vi "Get State.vi"(8 "error in (no error)":errorcluster, 11 "Dual Relay Bricklet in":refnum<class "Dual Relay Bricklet.lvclass">) -> (0 "error out":errorcluster, 1 "relay 2":bool, 2 "relay 1":bool, 3 "Dual Relay Bricklet out":refnum<class "Dual Relay Bricklet.lvclass">)   [LabVIEW 2011, in "Tinkerforge.lvlib" / "Dual Relay Bricklet.lvclass"]
doc: "This VI returns the state of both relays."
uses:
  Dual Relay Bricklet.lvclass
  Type Definitions/Relay States.ctl
  Device/Device.lvclass
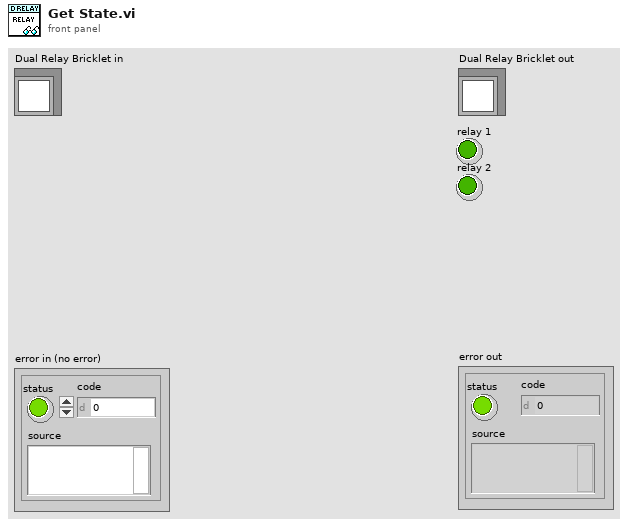
[diagram p1: front panel]
types:
  T1 = typedef "Tinkerforge.lvlib/Dual Relay Bricklet.lvclass/Relay States.ctl" = cluster{"relay 1":bool, "relay 2":bool}
  T2 = typedef "Tinkerforge.lvlib/IP Connection.lvclass/Answer.ctl" = cluster{"Request GUID":string, "Request Type":T3, "Sucessful":bool, "Data":variant, "Error":errorcluster}
  T3 = typedef "Tinkerforge.lvlib/IP Connection.lvclass/Request Type.ctl" = enum8{"Invalid", "Write"}
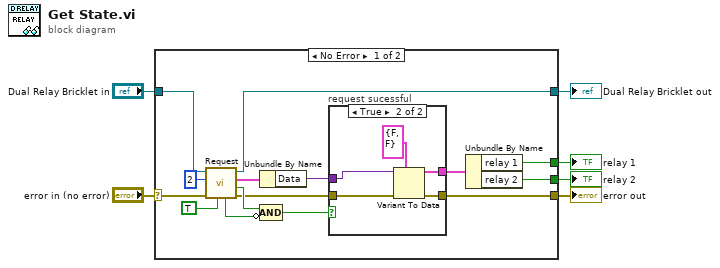
[diagram p0: block diagram]
diagram:
  n1 = case shown="No Error" "error in (no error)" {
    selector: "error in (no error)" -> [w21 w29]
    tunnel: [w10 w29] -> w5
    tunnel: [w19 w28] -> w3
    tunnel: "Dual Relay Bricklet in" -> [w20 w28]
    tunnel: [w8 _] -> w2
    tunnel: [w7 _] -> w1
    frame No Error {
      n2 = call "Request.vi"("Response"=TRUE, "error in (no error)"=w21, "Function ID"=u8 2, "Device in"=w20) -> ("error out"=w13:errorcluster, "Sucessful"=w15:bool, "Answer"=w12:T2, "Device out"=w19:refnum<class "Dual Relay Bricklet.lvclass">, "timed out"=w16:bool)  [unwired: 3 in]
      n3 = Unbundle By Name(w12) -> ("Data"=w11:variant)
      n4 = Compound Arithmetic op=AND(w15, invert w16) -> (w14:bool)
      n5 = case "request sucessful" shown="True" w14 {
        tunnel: w13 -> [w22 w27]
        tunnel: w11 -> [_ w25]
        tunnel: [_ w24] -> w9
        tunnel: [w22 w23] -> w10
        frame False {
        }
        frame True {
          n6 = Variant To Data(error in=w27, type=T1 {"relay 1"=FALSE, "relay 2"=FALSE} ("Data"), Variant=w25) -> (data=w24:T1, error out=w23:errorcluster)
        }
      }
      n7 = Unbundle By Name(w9) -> ("relay 1"=w8:bool, "relay 2"=w7:bool)
    }
    frame Error {
    }
  }
  "error out" <- w5
  "Dual Relay Bricklet out" <- w3
  "relay 1" <- w2
  "relay 2" <- w1
